vi "Program05.vi"() -> ()   [LabVIEW 2020]
panel:
  out "SR4":i32
  out "SR3":i32
  out "SR2":i32
  out "SR1":i32
  out "Wynik":i32
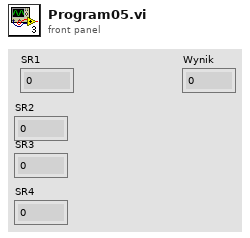
[diagram p1: front panel]
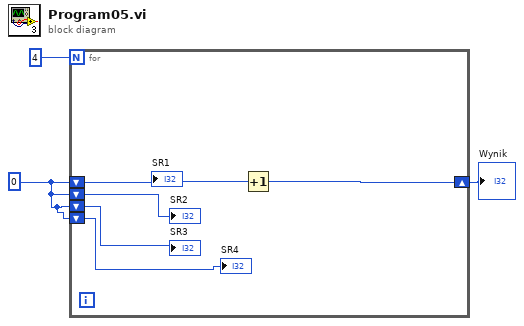
[diagram p0: block diagram]
diagram:
  w1 = 0
  n1 = for {
    N: 4 -> [_]
    shift-right: [w8] -> w2
    shift-left: w1 -> [w7]
    shift-left: w1 -> [w6]
    shift-left: w1 -> [w5]
    shift-left: w1 -> [w4]
    n2 = Increment(x=w7) -> (x+1=w8:i32)
    "SR1" <- w7
    "SR2" <- w6
    "SR3" <- w5
    "SR4" <- w4
  }
  "Wynik" <- w2
